vi "Main.vi"() -> ()   [LabVIEW 2015]
uses:
  TypeDefs/Queue Data.ctl
  FGV/Timer Actions.ctl
  SubVIs/App Data.vi
  SubVIs/App Strings.vi
  Laboratorium 3/Weather Warnings/Global 3.vi
panel:
  in  "Period [s]":dbl
  in  "Device name":tag="myDAQ1"
  out "Time Elapsed":dbl format="%<%M:%S>t"
  out "Status":string
  in  "Time [ms]":dbl
  in  "Frequency":dbl
  in  "Stop Button":bool
  in  "Acquire Button":bool
  out "Waveform Graph":dbl[](graph)
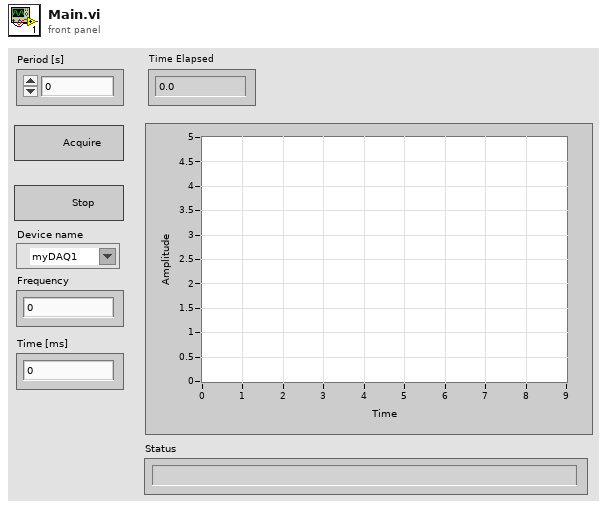
[diagram p1: front panel]
types:
  T1 = typedef "Timer Actions.ctl" = enum16{"Reset", "Get"}
  T2 = typedef "Queue Data.ctl" = cluster{"Action":string}
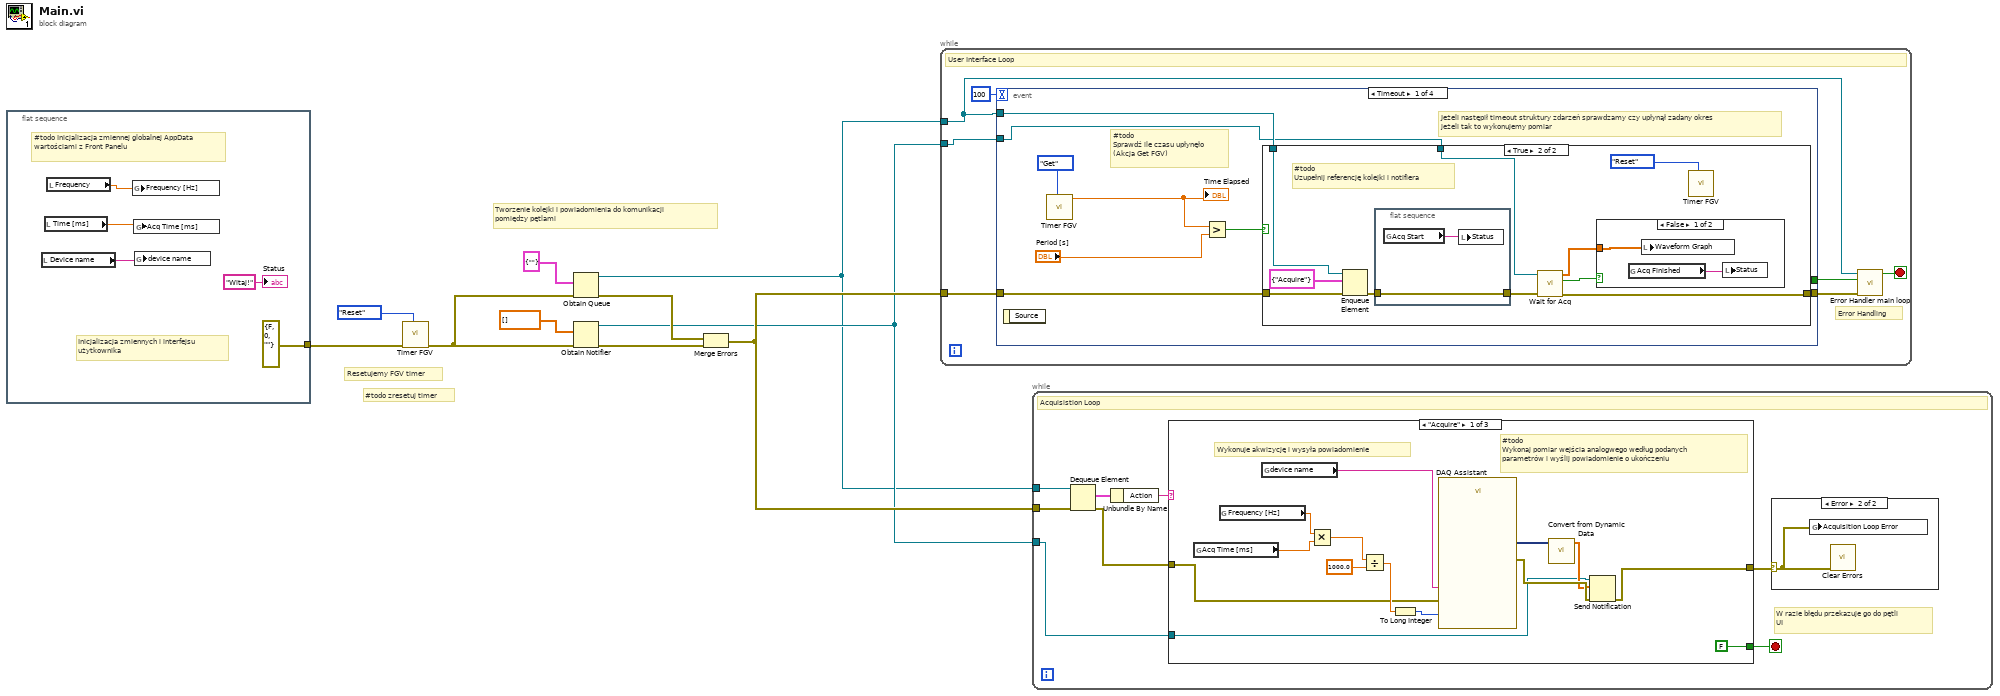
[diagram p0: block diagram]
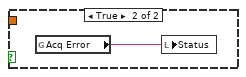
[diagram p3: hidden frame]
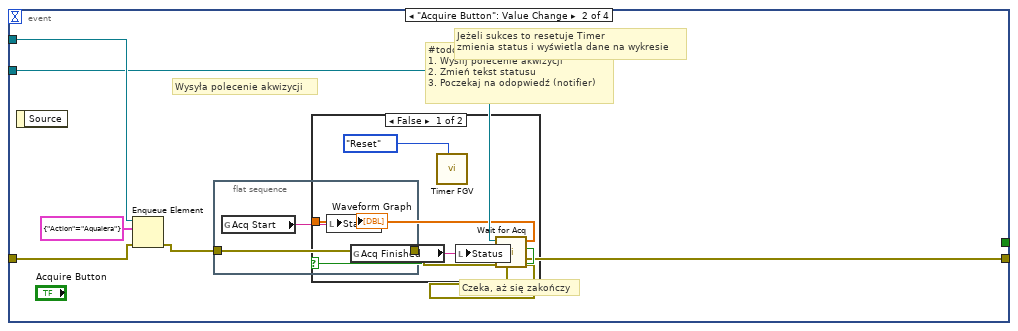
[diagram p4: hidden frame]
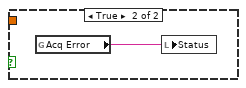
[diagram p5: hidden frame]
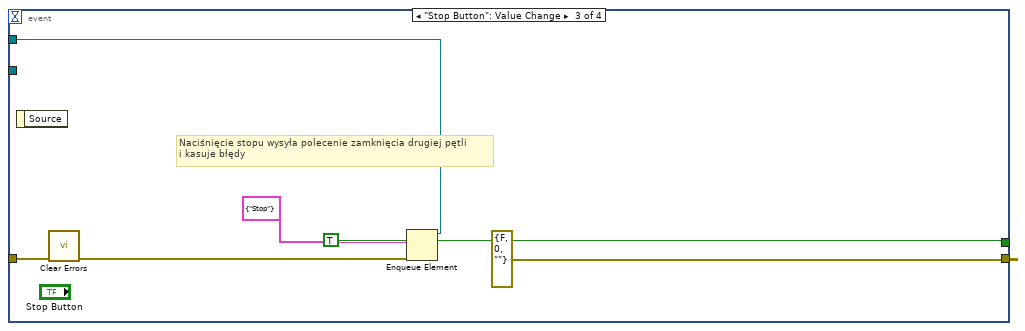
[diagram p6: hidden frame]
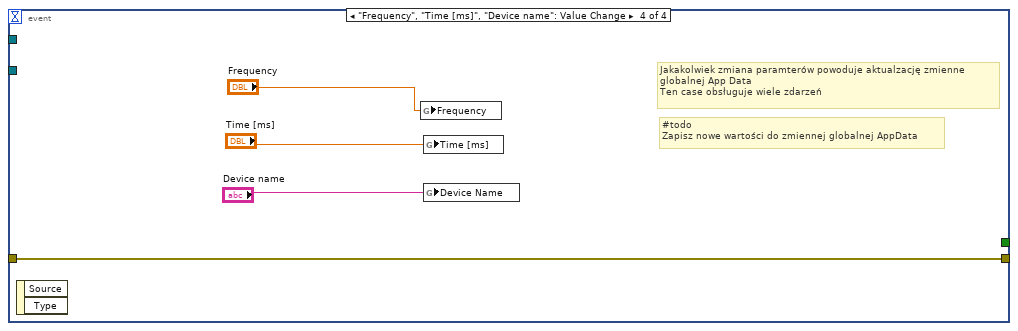
[diagram p7: hidden frame]
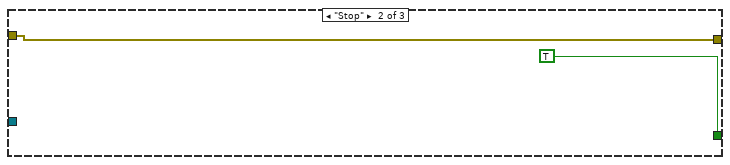
[diagram p9: hidden frame]
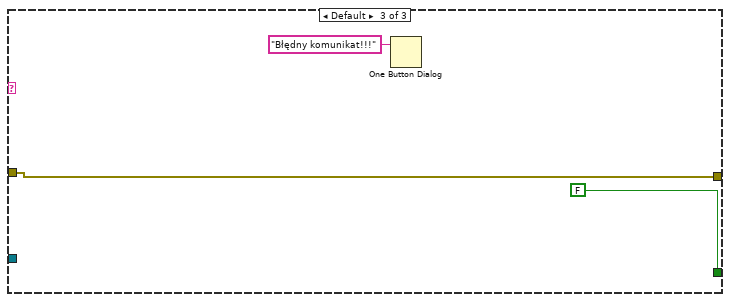
[diagram p10: hidden frame]
diagram:
  # "#todo zresetuj timer"
  # "Resetujemy FGV timer"
  # "Tworzenie kolejki i powiadomienia do komunikacji \npomiędzy pętlami"
  n1 = flat-sequence {
    tunnel: [errorcluster {"status"=FALSE, "code"=0, "source"=""} ("error constant")] -> w3
    frame #0 {
      # "#todo Inicjalizacja zmiennej globalnej AppData wartościami z Front Panelu"
      # "Inicjalizacja zmiennych i interfejsu \nużytkownika"
      n2 = local read "Device name"() -> (w11:tag)
      n3 = local read "Time [ms]"() -> (w12:dbl)
      n4 = local read "Frequency"() -> (w13:dbl)
      n5 = global write "App Data.vi" "Frequency [Hz]"(w13) -> ()
      n6 = global write "App Data.vi" "Acq Time [ms]"(w12) -> ()
      n7 = global write "App Data.vi" "device name"(w11) -> ()
      "Status" <- "Witaj!" ("Status")
    }
  }
  n8 = call "Timer FGV.vi"("Action"=Timer_Actions."Reset", "error in (no error)"=w3) -> ("error out"=w2:errorcluster)  [unwired: 8 in, 1 out]
  n9 = Obtain Queue(element data type=T2 {"Action"=""}, error in (no error)=w2) -> (queue out=w4:refnum<queue>, error out=w9:errorcluster)  [unwired: 3 in, 1 out]
  n10 = Obtain Notifier(notification data type=dbl[] [], error in (no error)=w2) -> (notifier out=w5:refnum<notifier>, error out=w7:errorcluster)  [unwired: 2 in, 1 out]
  n11 = Merge Errors(w9, w7) -> (w6:errorcluster)
  n12 = while {
    tunnel: w6 -> [w21]
    tunnel: w4 -> [w17]
    tunnel: w5 -> [w16]
    stop <- w18 stop-if-true
    # "Error Handling"
    # "User Interface Loop"
    n13 = event shown="[0] Timeout" {
      selector: _ -> [_ _ _ _]
      dyn-events: _ -> [_ _ _ _]
      timeout: 100 -> [_ _ _ _]
      tunnel: w21 -> [w28 w55 w64 w71]
      tunnel: [w27 w47 errorcluster {"status"=FALSE, "code"=0, "source"=""} ("error constant") w71] -> w19
      tunnel: [_ _ TRUE _] -> w20
      tunnel: w17 -> [w26 w54 w62 _]
      tunnel: w16 -> [w25 w50 _ _]
      event Timeout {
        # "#todo\nSprawdź ile czasu upłynęło\n(Akcja Get FGV)"
        # "Jeżeli następił timeout struktury zdarzeń sprawdzamy czy upłynął zadany okres \njeżeli tak to wykonujemy pomiar"
        n14 = event-data() -> ()  [unwired: 1 in, 1 out]
        n15 = call "Timer FGV.vi"("Action"=Timer_Actions."Get") -> ("Elapsed Time"=w23:dbl)  [unwired: 9 in, 1 out]
        "Time Elapsed" <- w23
        n16 = Greater?(x=w23, y="Period [s]") -> (0:w29:bool)
        n17 = case shown="True" w29 {
          tunnel: w28 -> [w31 w41]
          tunnel: [w31 w34] -> w27
          tunnel: w26 -> [_ w33]
          tunnel: w25 -> [_ w32]
          frame False {
          }
          frame True {
            # "#todo\nUzupełnij referencję kolejki i notifiera"
            n18 = Enqueue Element(queue=w33, element=T2 {"Action"="Acquire"}, error in (no error)=w41) -> (error out=w39:errorcluster)  [unwired: 1 in, 2 out]
            n19 = flat-sequence {
              tunnel: w39 -> [w45]
              tunnel: [w45] -> w38
              frame #0 {
                n20 = global read "App Strings.vi" "Acq Start"() -> (w46:string)
                n21 = local write "Status"(w46) -> ()
              }
            }
            n22 = call "Wait for Acq.vi"("error in (no error)"=w38, "Notifier in"=w32) -> ("error out"=w34:errorcluster, "timed out?"=w35:bool, "Array"=w37:dbl[])  [unwired: 7 in]
            n23 = case shown="False" w35 {
              tunnel: w37 -> [w42 _]
              frame False {
                n24 = global read "App Strings.vi" "Acq Finished"() -> (w43:string)
                n25 = local write "Waveform Graph"(w42) -> ()
                n26 = local write "Status"(w43) -> ()
              }
              frame True {
                n27 = global read "App Strings.vi" "Acq Error"() -> (w44:string)
                n28 = local write "Status"(w44) -> ()
              }
            }
            n29 = call "Timer FGV.vi"("Action"=Timer_Actions."Reset") -> ()  [unwired: 9 in, 2 out]
          }
        }
      }
      event "Acquire Button": Value Change {
        # "#todo\n1. Wyślij polecenie akwizycji\n2. Zmień tekst statusu\n3. Poczekaj na odopwiedź (notifier)"
        # "Jeżeli sukces to resetuje Timer\nzmienia status i wyświetla dane na wykresie"
        # "Czeka, aż się zakończy"
        # "Wysyła polecenie akwizycji"
        n30 = event-data() -> ()  [unwired: 1 in, 1 out]
        n31 = Enqueue Element(queue=w54, element=T2 {"Action"="Aquaiera"}, error in (no error)=w55) -> (error out=w52:errorcluster)  [unwired: 1 in, 2 out]
        n32 = flat-sequence {
          tunnel: w52 -> [w56]
          tunnel: [w56] -> w51
          frame #0 {
            n33 = global read "App Strings.vi" "Acq Start"() -> (w57:string)
            n34 = local write "Status"(w57) -> ()
          }
        }
        n35 = call "Wait for Acq.vi"("error in (no error)"=w51, "Notifier in"=w50) -> ("error out"=w47:errorcluster, "timed out?"=w49:bool, "Array"=w48:dbl[])  [unwired: 7 in]
        n36 = case shown="False" w49 {
          tunnel: w48 -> [w58 _]
          frame False {
            n37 = global read "App Strings.vi" "Acq Finished"() -> (w60:string)
            n38 = call "Timer FGV.vi"("Action"=Timer_Actions."Reset") -> ()  [unwired: 9 in, 2 out]
            n39 = local write "Status"(w60) -> ()
            "Waveform Graph" <- w58
          }
          frame True {
            n40 = global read "App Strings.vi" "Acq Error"() -> (w61:string)
            n41 = local write "Status"(w61) -> ()
          }
        }
      }
      event "Stop Button": Value Change {
        # "Naciśnięcie stopu wysyła polecenie zamknięcia drugiej pętli\ni kasuje błędy"
        n42 = event-data() -> ()  [unwired: 1 in, 1 out]
        n43 = call <vilib>:"Clear Errors.vi"("error in (no error)"=w64) -> ("error out"=w63:errorcluster)  [unwired: 5 in, 1 out]
        n44 = Enqueue Element(queue=w62, element=T2 {"Action"="Stop"}, error in (no error)=w63) -> ()  [unwired: 1 in, 3 out]
      }
      event "Frequency", "Time [ms]", "Device name": Value Change {
        # "#todo \nZapisz nowe wartości do zmiennej globalnej AppData"
        # "Jakakolwiek zmiana paramterów powoduje aktualzację zmienne \nglobalnej App Data\nTen case obsługuje wiele zdarzeń"
        n45 = event-data() -> ()  [unwired: 1 in, 2 out]
        n46 = global write "Global 3.vi" "Frequency"("Frequency") -> ()
        n47 = global write "Global 3.vi" "Time [ms]"("Time [ms]") -> ()
        n48 = global write "Global 3.vi" "Device Name"("Device name") -> ()
      }
    }
    n49 = call "Error Handler main loop.vi"("error in (no error)"=w19, "Exit?"=w20, "Queue in"=w17) -> ("Exit?"=w18:bool)  [unwired: 8 in]
  }
  n50 = while {
    tunnel: w6 -> [w77]
    tunnel: w4 -> [w73]
    tunnel: w5 -> [w72]
    stop <- w75 stop-if-true
    # "W razie błędu przekazuje go do pętli\nUI"
    # "Acquisistion Loop"
    n51 = Dequeue Element(queue=w73, error in (no error)=w77) -> (element=w79:T2, error out=w76:errorcluster)  [unwired: 1 in, 2 out]
    n52 = Unbundle By Name(w79) -> ("Action"=w78:string)
    n53 = case shown="\"Acquire\"" w78 {
      tunnel: w76 -> [w86 w95 w98]
      tunnel: [FALSE TRUE FALSE] -> w75
      tunnel: [w84 w95 w98] -> w74
      tunnel: w72 -> [w81 _ _]
      frame "Acquire" {
        # "#todo\nWykonaj pomiar wejścia analogwego według podanych \nparametrów i wyślij powiadomienie o ukończeniu"
        # "Wykonuje akwizycję i wysyła powiadomienie"
        n54 = global read "App Data.vi" "Acq Time [ms]"() -> (w91:dbl)
        n55 = global read "App Data.vi" "Frequency [Hz]"() -> (w92:dbl)
        n56 = global read "App Data.vi" "device name"() -> (w93:tag)
        n57 = Multiply(x=w92, y=w91) -> (x*y=w90:dbl)
        n58 = Divide(x=w90, y=1000.0) -> (x/y=w87:dbl)
        n59 = To Long Integer(number=w87) -> (32bit integer=w88:i32)
        n60 = call "DAQ Assistant"("number of samples"=w88, "error in"=w86, "device name"=w93) -> ("data"=w83:dynamicdata, "error out"=w85:errorcluster)  [unwired: 14 in, 1 out]
        n61 = call "Convert from Dynamic Data"("Dynamic Data Type"=w83) -> ("Array"=w82:dbl[])  [unwired: 3 in]
        n62 = Send Notification(notification=w82, notifier=w81, error in (no error)=w85) -> (error out=w84:errorcluster)  [unwired: 1 out]
      }
      frame "Stop" {
      }
      frame Default {
        n63 = One Button Dialog(message="Błędny komunikat!!!") -> ()  [unwired: 1 in, 1 out]
      }
    }
    n64 = case shown="Error" w74 {
      selector: w74 -> [_ w80]
      frame No Error {
      }
      frame Error {
        n65 = global write "App Data.vi" "Acquisition Loop Error"(w80) -> ()
        n66 = call <vilib>:"Clear Errors.vi"("error in (no error)"=w80) -> ()  [unwired: 5 in, 2 out]
      }
    }
  }
